vi "Write Trig Resolution.vi"(8 "error in (no error)":errorcluster, 10 "Trig Resolution":u32 caption="Trig Resolution, ms", 11 "TRIG Next Acq Request in":refnum<class "TRIG Next Acq Request.lvclass">) -> (0 "error out":errorcluster, 3 "TRIG Next Acq Request out":refnum<class "TRIG Next Acq Request.lvclass">)   [LabVIEW 2019, in "Trig Process.lvlib" / "TRIG Next Acq Request.lvclass"]
uses:
  TRIG Next Acq Request.lvclass
  TRIG Next Acq Request.lvclass/TRIG Next Acq Request.ctl
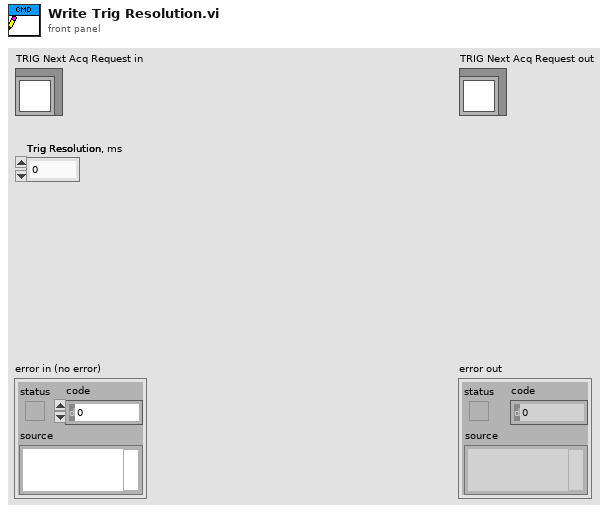
[diagram p1: front panel]
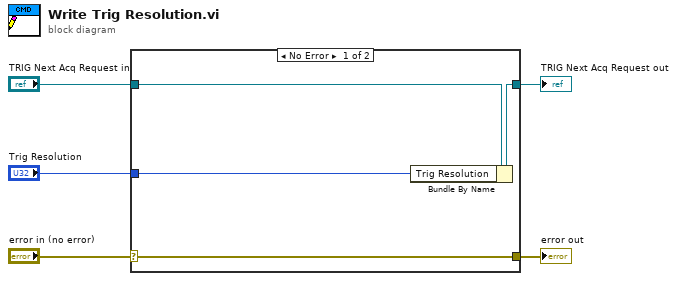
[diagram p0: block diagram]
diagram:
  n1 = case shown="No Error" "error in (no error)" {
    selector: "error in (no error)" -> [w9 w10]
    tunnel: [w9 w10] -> w4
    tunnel: [w7 w11] -> w2
    tunnel: "TRIG Next Acq Request in" -> [w8 w11]
    tunnel: "Trig Resolution" -> [w6 _]
    frame No Error {
      n2 = Bundle By Name(cluster=w8, "Trig Resolution"=w6) -> (w7:refnum<class "TRIG Next Acq Request.lvclass">)
    }
    frame Error {
    }
  }
  "error out" <- w4
  "TRIG Next Acq Request out" <- w2
